vi "AlliGator Load I-m-phi Dataset.vi"(5 "Image Type":string="Image", 7 "Bkgd Image Subtraction?":bool, 8 "error in (no error)":errorcluster, 9 "Control References":T1, 10 "Folder Path":path, 11 "AlliGator IV DVR in":refnum<data-value>) -> (0 "error out":errorcluster, 2 "Folder Path (dup)":path, 3 "AlliGator IV DVR out":refnum<data-value>, 4 "Result String":string)   [LabVIEW 2021, in "AlliGator Files.lvlib"]
doc: "Loads a FLI dataset comprised of an intensity and phase image (FLIMBox)."
uses:
  AlliGator Files.lvlib
  Internal Variables/AlliGator Internal Variables v2.ctl
  <vilib>/vision/Image Controls.llb/IMAQ Image.ctl
  Internal Variables/AlliGator Gate Image Set.ctl
  AlliGator FLI Dataset Type.ctl
  AlliGator Data Series Type.ctl
  Dual-Channel Datasets/AlliGator Dataset Channel.ctl
  Settings/AlliGator Gate Arithmetic.ctl
  Source Image/AlliGator Displayed Image.ctl
  Image/Named ROI Description.ctl
  Phasor Graph/AlliGator Decay Metadata v3.ctl
  Decay Analysis/Decay Preprocessing/AlliGator Decay Background Subtraction Info.ctl
  Decay Analysis/Decay Preprocessing/AlliGator Baseline Subtraction Method.ctl
  Graphs/XY Graph/XY Graph Plot Shift Parameters.ctl
  Graphs/XY Graph/XY Graph Plot Shift Method.ctl
  Decay Analysis/Decay Preprocessing/AlliGator Decay Extrapolation Parameters.ctl
  Phasor/Calibration Phasor (m, phi).ctl
  Phasor/Phasor Reference Series.ctl
  Phasor/Phasor Calibration Map v2.ctl
  Phasor/Phasor (g, s).ctl
  Phasor Graph/AlliGator Raw Phasor Plot Data v5.ctl
  Phasor/Phasor Standard Deviation Options.ctl
  Phasor Plot/AlliGator Phasor Multi-Harmonic Data.ctl
  Phasor/Phasor Harmonic Data.ctl
  Decay Fit Parameter Map/AlliGator Decay Fit Options & Parameters v4.ctl
  Fits/IRF(X)PSED/Decay Fit Options v4.ctl
  Fits/Decay Convolution/Decay Model.ctl
  Fits/Residual Type.ctl
  Fits/IRF(X)PSED/Fit Weights Type v2.ctl
  Fits/Non-linear Fitting Method v2.ctl
  Fits/Fit Calculation Method.ctl
  Fits/Non-linear Fitting Algorithm.ctl
  Decay Analysis/Decay Fit/AlliGator Decay Fit Parameter Constraints 2.ctl
  Fits/IRF(X)PSED/Decay Fit Parameters In List.ctl
  Fits/IRF(X)PSED/MLE Baseline Offset Type.ctl
  Decay Analysis/Decay Preprocessing/AlliGator Decay Preprocessing Parameters.ctl
  Fits/IRF(X)PSED/Decay Fit Parameters & Derived Quantities List v2.ctl
  Fits/IRF(X)PSED/Decay Fit Result Constraint.ctl
  Decay Fit Parameter Map/AlliGator Parameter Maps Data.ctl
  GUI/AlliGator Dataset Ctrl Refnums.ctl
  AlliGator After Loading Dataset Information.ctl
  AlliGator ICCD-specific Information.ctl
  AlliGator I-m-phi Component List.ctl
  089290e1-c93f-4b42-a3f3-b2d44885c075.vi
  Arrays/n x n Kernel Convolution (SGL).vi
  Arrays/n x n Smoothen Array (SGL) v3.vi
  Arrays/n x n Kernel Convolution (SGL).vi/d0ebc029-cbaa-4c82-a58c-923c59c440da.vi
  Arrays/n x n Kernel Convolution (SGL).vi/b80d5e79-a0c8-46e2-aba9-3d60e0093a16.vi
  <vilib>/Analysis/2dsp.llb/Convolution.vi
  <vilib>/Analysis/2dsp.llb/2D Convolution (DBL).vi
  Arrays/Truncate Kernel.vi
  Arrays/Replace NaN by 0 (2D SGL).vi
  Arrays/n x n Smoothen Array (SGL) v3.vi/d0ebc029-cbaa-4c82-a58c-923c59c440da.vi
  Arrays/n x n Smoothen Array (SGL) v3.vi/b80d5e79-a0c8-46e2-aba9-3d60e0093a16.vi
  Arrays/Replace NaN by 0 (2D SGL).vi/df975b44-f6c5-4554-af30-980613d33749.vi
  Time/High Resolution Timing.vi
  Arrays/Compute n x n Kernel (SGL).vi
  <vilib>/Utility/error.llb/Simple Error Handler.vi
  <vilib>/Utility/error.llb/Error Cluster From Error Code.vi
  <vilib>/ErrorRing/Error Ring.xnode
  Image/Image.lvlib
  Source Image/AlliGator Source Image.lvlib
  GUI/AlliGator GUI.lvlib
  GUI/GUI.lvlib
  Boolean/Boolean.lvlib
  Error/Error.lvlib
  Arrays/Arrays.lvlib
  Strings/Strings.lvlib
  Internal Variables/AlliGator Internal Variables.lvlib
  Phasor/Phasor.lvlib
  Decay Analysis/Decay Preprocessing/AlliGator Decay Preprocessing.lvlib
  Graphs/XY Graph/XY Graph Add-Ons.lvlib
  Phasor Graph/AlliGator Phasor Graph.lvlib
  Phasor Plot/AlliGator Phasor Plot.lvlib
  Fits/Fits.lvlib
  Decay Analysis/Decay Fit/AlliGator Decay Fit.lvlib
  Settings/AlliGator Settings.lvlib
  Dual-Channel Datasets/AlliGator Dual-Channel Datasets.lvlib
  Decay Fit Parameter Map/AlliGator Decay Fit Parameter Map.lvlib
panel:
  out "# disposed images":i32
  out "# created images":i32
  # "see the AlliGator License on the block diagram (Ctrl+E or Window:Show Block Diagram)"
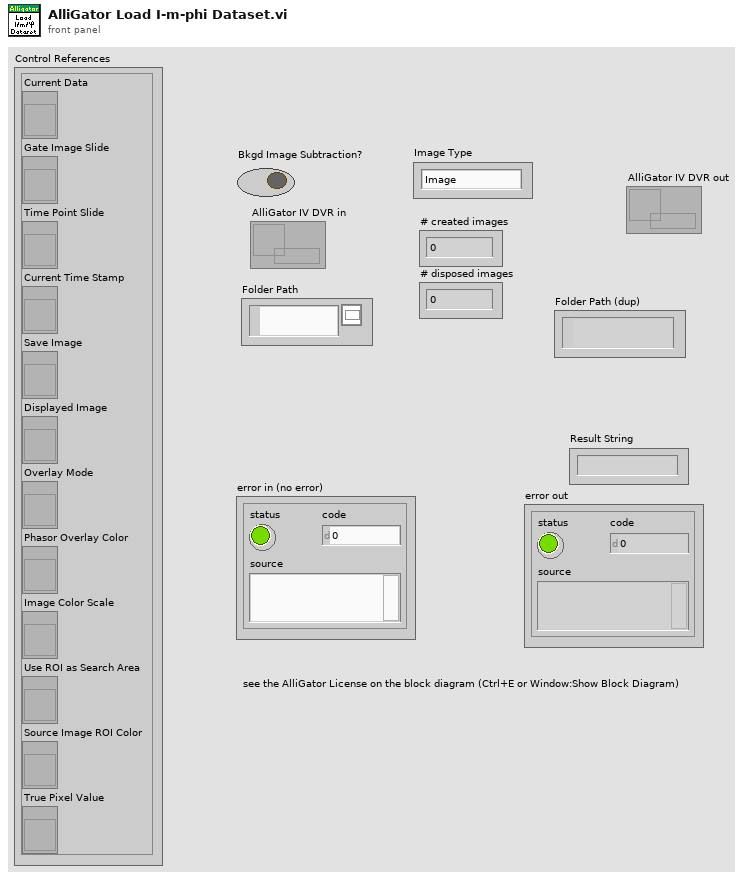
[diagram p1: front panel]
types:
  T1 = typedef "AlliGator GUI.lvlib/AlliGator Dataset Ctrl Refnums.ctl" = cluster{"Current Data":refnum<vi>, "Gate Image Slide":refnum<vi>, "Time Point Slide":refnum<vi>, "Current Time Stamp":refnum<vi>, "Save Image":refnum<vi>, "Displayed Image":refnum<vi>, "Overlay Mode":refnum<vi>, "Phasor Overlay Color":refnum<vi>, "Image Color Scale":refnum<vi>, "Use ROI as Search Area":refnum<vi>, "Source Image ROI Color":refnum<vi>, "True Pixel Value":refnum<vi>}
  T2 = typedef "AlliGator Files.lvlib/AlliGator After Loading Dataset Information.ctl" = cluster{"Nanotime Gate Separation":dbl[unit], "Gate Width":dbl[unit], "Laser Period":dbl[unit], "Data Description":string, "# Pixel X":i32, "# Pixel Y":i32, "Gates to Use":cluster{"Start":u32, "End":u32}, "Gate Step":i32, "SYNC Period":dbl[unit], "X Binning":i32, "Y Binning":i32, "Gates to":bool, "Metadata":string, "Gate Image Exposure":dbl[unit], "Gate Image Integration":dbl[unit], "Macrotime Gate Separation":dbl[unit], "ICCD-specific Information":T3}
  T3 = typedef "AlliGator Files.lvlib/AlliGator ICCD-specific Information.ctl" = cluster{"V MCP":dbl[unit], "X Hardware Binning":dbl, "Y Hardware Binning":dbl, "Gate Image Integration":dbl[unit], "Laser Power":dbl[unit]}
  T4 = typedef "AlliGator Files.lvlib/AlliGator FLI Dataset Type.ctl" = enum16{"HDF5 FLI Dataset", "Gate Image Folder", ".sdt FLI Dataset (Becker & Hickl)", ".ptu FLI Dataset (PicoQuant)", "SS1 FLI Dataset", "SS2 FLI Dataset", "I/m/phi Dataset", ".bin FLI Dataset (PicoQuant Binned)", ".bin FLI Dataset (Piccolo Binned)", ".mat FLI Dataset"}
  T5 = typedef "AlliGator Internal Variables.lvlib/AlliGator Gate Image Set.ctl" = cluster{"SGL Image Max":T6, "SGL Image Sum":T6, "SGL Gate Images":T6[], "SGL Image Min":T6}
  T6 = typedef "IMAQ Image.ctl" = refnum<image>
  T7 = typedef "AlliGator Files.lvlib/AlliGator I-m-phi Component List.ctl" = enum16{"Intensity", "g", "s"}
  T8 = typedef "FLIMBox.lvlib/FLIMbox Data.ctl" = cluster{"Software":string, "Base Frequency":dbl[unit], "X Size":i32, "Y Size":i32, "Metadata":string, "Intensity":sgl[][], "Harmonic Number":u8, "Harmonic Orders":u8[], "Harmonic Data":T9[], "File Version":string}
  T9 = typedef "FLIMBox.lvlib/FLIMbox Harmonic Data.ctl" = cluster{"Modulus":sgl[][], "Phase":sgl[][], "Harmonic Order":u8}
  T10 = typedef "AlliGator Source Image.lvlib/AlliGator Image Loading Options.ctl" = cluster{"Pixel Well Capacity":u32, "Pile-up Correction":bool, "Gate Step":i32, "Image Smoothing Options":T11, "Gates to Skip":T14, "File Background Subtraction":bool, "Background File Path":path, "Image Binning Options":T15, "# Gates":u32, "Gates to Keep":T16, "Define Gates to":bool, "Hot Pixel Removal":T17, "Dataset Scaling Factor":dbl, "Image Pre-processing Steps":T18[]}
  T11 = typedef "AlliGator Settings.lvlib/AlliGator Image Smoothing Options.ctl" = cluster{"Use Image Smoothing":bool, "Kernel Type":T12, "Bin":i32, "Algorithm":T13}
  T12 = typedef "Arrays.lvlib/Kernel Type.ctl" = enum16{"Uniform", "Bilinear", "Gaussian"}
  T13 = typedef "Arrays.lvlib/Smoothing Algorithm.ctl" = enum16{"Rapid", "Thorough"}
  T14 = typedef "AlliGator Settings.lvlib/AlliGator Background Subtraction Parameters.ctl" = cluster{"Start":u32, "End":u32}
  T15 = typedef "AlliGator Source Image.lvlib/AlliGator Image Binning Options.ctl" = cluster{"Use Image Binning":bool, "X Bin":i32, "Y Bin":i32}
  T16 = typedef "AlliGator Settings.lvlib/AlliGator Gates to Keep.ctl" = cluster{"First":u32, "Last":u32}
  T17 = typedef "SwissSPAD Live.lvlib/SwissSPAD Live_Image Display Options.ctl" = cluster{"Remove Screamers":bool, "Delta":sgl, "Equalize Histogram":bool, "Percentile":sgl, "Hot Pixel Mask Image":path, "Use Hot Pixel Mask":bool}
  T18 = typedef "AlliGator Files.lvlib/AlliGator Image Pre-processing Step.ctl" = enum16{"Remove Screamers", "Pile-up Correction", "Binning", "Smoothing", "Rescaling", "Dead Left Column Correction"}
  T19 = typedef "AlliGator Internal Variables.lvlib/AlliGator Internal Variables v2.ctl" = cluster{"----------------------------- Images -----------------------------":u8, "Displayed Image":T6, "White Light Image":T6, "Mask Image":T6, "ROI Mask Image":T6, "Current Dataset Images 1":T5, "Background Dataset Images 1":T5, "Current Dataset Images 2":T5, "Background Dataset Images 2":T5, "Current Dataset Arithmetic Images":T5, "Accumulated Dataset Images 1":T5, "Accumulated Dataset Images 2":T5, "Accumulated Dataset Arithmetic Images":T5, "----------------------------- File Paths -----------------------------":u8, "Phasor Plot Image":T6, "Decay Fit Parameter Map Image":T6, "Parameter Map Image":T6, "Single Data Point Path":path, "White Light Image Path":path, "Mask Image Path":path, "Time-Series Folder":path, "[Time-Series Paths]":path[], "----------------------------- FLI Dataset -----------------------------":u8, "Current Dataset":i32, "Single Dataset Type":T4, "Current Folder":string, "AlliGator Data Series Type":T20, "# Datasets":i32, "Dual-Channel Dataset":bool, "Selected Channel Name":string, "Dataset Channel":T21, "Channel Arithmetic":T22, "Dual-Channel Background Dataset":bool, "Background Channel":T21, "Dual-Channel Accumulated Dataset":bool, "Start Time":dbl, "[Time-Series Timestamps]":dbl[], "[Intensity Corrections]":dbl[], "Time Series Script":bool, "Type of Displayed Image":T23, "Gate Image Slide":u16, "# Gates":i32, "ROIs":T24[], "----------------------------- Decays -----------------------------":u8, "ROI Decay":cluster{"t Array":dbl[], "I Array":dbl[]}, "Valid Decay":bool, "Decay  Metadata":T26, "Reference Decay Plot Name":string, "Reference Decay":cluster{"t Array":dbl[], "I Array":dbl[]}, "Decay Shift Plot":cluster{"Time Stamps":dbl[], "Decay Shifts":dbl[]}, "[Decays Max Values]":sgl[], "[Decays Min Values]":sgl[], "----------------------------- Calibration -----------------------------":u8, "Calibration Phasor":T32, "Calibration Phasor Series":T33, "Phasor Calibration Map":T34, "Calibration Map MD5 Digest":string, "----------------------------- Phasor Graph -----------------------------":u8, "Last Raw Phasor":T35, "Last Calibrated Phasor":T35, "Last Calibrated Phasor SDV":T35, "Phasor Graph:Phasor Plot":cluster{"g Array":dbl[], "s Array":dbl[]}, "Phasor Graph:Phasor SDV Plot":cluster{"g Array":dbl[], "s Array":dbl[]}, "[Phasor Graph:Raw Phasor Plots]":T36[], "Phasor Plot locked to Ref 1":i32, "[Phasor Plot(s) locked to Ref 1]":i32[], "[Phasor Plot(s) locked to Ref 2]":i32[], "[Pixel Phasors]":T35[], "----------------------------- Phasor Plot -----------------------------":u8, "[[Sum Image]]":dbl[][], "[[CSG Phasors]]":csg[][], "[[Valid Pixel?]]":bool[][], "[[Phasor Ratios]]":dbl[][], "[[Average Lifetimes]]":dbl[][], "Amplitude Weighted Average Lifetime":bool, "I/m/phi Dataset":cluster{"I/m/phi Dataset?":bool, "Base Frequency":dbl[unit], "Harmonic Orders":u8[]}, "Multi Phasor Plot Data":T38, "----------------------------- Decay Fit Parameter Map -----------------------------":u8, "Decay Fit Options & Parameters":T40, "Fit Options: Decay Preprocessing Parameters":T51, "Fit Options: Reference Decay":cluster{"t Array":dbl[], "I Array":dbl[]}, "Is Full Image Parameters Map":bool, "Is Single-Pixels Parameters Map":bool, "NLSF Parameters Map X Resolution":i32, "NLSF Parameters Map Y Resolution":i32, "[Single Decay Fit Parameters]":dbl[], "Fit Model":T42, "[[Multiple Decays Fit Parameters]]":dbl[][], "[[Multiple Decays Fit Parameter SDVs]]":dbl[][], "[[IRFs]]":dbl[][], "[ROI Descriptors]":T25[], "IRF Array Time Axis":dbl[], "Decay Array Time Axis":dbl[], "[Decay Fit Parameter Names]":T52[], "[Decay Sum]":dbl[], "Array of Decay Fit Result Constraints":T53[], "Selected ROIs Array":bool[], "----------------------------- Parameter Maps -----------------------------":u8, "[Map Set Names]":string[], "[Parameter Maps]":T54[], "[[User-defined Quantities]]":dbl[][], "User-defined Quantity":string}
  T20 = typedef "AlliGator Files.lvlib/AlliGator Data Series Type.ctl" = enum16{"Not a Supported Series", "Gate Images Folder Series", "SwissSPAD 2 Dataset Series", "B&H FLI Dataset Series", "PicoQuant PTU FLI Dataset Series", "PicoQuant BIN FLI Dataset Series", "Piccolo hist BIN FLI Dataset Series", "HDF5 FLI Dataset Series"}
  T21 = typedef "AlliGator Dual-Channel Datasets.lvlib/AlliGator Dataset Channel.ctl" = enum16{"G2", "INT"}
  T22 = typedef "AlliGator Settings.lvlib/AlliGator Gate Arithmetic.ctl" = enum16{"None", "INT-G2", "G2/INT*<INT>", "(1 - G2/INT)*<INT>"}
  T23 = typedef "AlliGator Source Image.lvlib/AlliGator Displayed Image.ctl" = enum16{"Single Gate", "Sum of All Gates", "Max of All Gates", "Min of All Gates", "-", "White Ligth Image", "Mask Image"}
  T24 = typedef "Image.lvlib/Named ROI Description.ctl" = cluster{"ROI Descriptor":T25, "ROI Name":string, "Overlay Color":u32}
  T25 = typedef "ROI Descriptor" = cluster{"Global Rectangle":i32[], "Contours":cluster{"ID":enum32{"External", "Internal"}, "Type":u32, "Coordinates":i32[]}[]}
  T26 = typedef "AlliGator Phasor Graph.lvlib/AlliGator Decay Metadata v3.ctl" = cluster{"ROI Descriptor":T25, "ROI Center":cluster{"X":i32, "Y":i32}, "Decay Background Subtraction Info":T27, "Decay Reverted":bool, "Decay Smoothened":bool, "Decay Straightened":bool, "Fitted Tau (Decay Straightening)":dbl, "Decay Shift Parameters":T29, "Decay Shifted":bool, "Decay Extrapolated":bool, "Decay Extrapolation Parameters":T31, "Decay Normalized":bool, "Fold Decay":bool, "# Folds":u32}
  T27 = typedef "AlliGator Decay Preprocessing.lvlib/AlliGator Decay Background Subtraction Info.ctl" = cluster{"Laser Period":dbl[unit], "Gate Duration":dbl[unit], "Baseline Subtraction Method":T28, "Background Definition Range":cluster{"Min Gate":dbl[unit], "Max Gate":dbl[unit]}, "Total Intensity w/o Bkgd Subtraction":dbl, "Bkgd-subtracted Intensity (exp)":dbl, "# Data Points":i32, "Background/Gate":dbl, "Fitted Lifetime":dbl[unit], "Bkgd-subtracted Intensity (theo)":dbl}
  T28 = typedef "AlliGator Decay Preprocessing.lvlib/AlliGator Baseline Subtraction Method.ctl" = enum16{"Mean", "Min", "Square Gated Single-Exponential", "File", "Constant"}
  T29 = typedef "XY Graph Add-Ons.lvlib/XY Graph Plot Shift Parameters.ctl" = cluster{"Type":T30, "Shift":dbl[unit], "Threshold":dbl, "Rotate":bool}
  T30 = typedef "XY Graph Add-Ons.lvlib/XY Graph Plot Shift Method.ctl" = enum16{"Default", "CFD", "Threshold", "Cross-Correlation"}
  T31 = typedef "AlliGator Decay Preprocessing.lvlib/AlliGator Decay Extrapolation Parameters.ctl" = cluster{"Additional Points":u32, "Head Fraction":dbl, "Fitted Tau":dbl, "Use Periodicity":bool, "Use Cursors":bool, "Tail Fraction":dbl}
  T32 = typedef "Phasor.lvlib/Calibration Phasor (m, phi).ctl" = cluster{"m":dbl, "phi":dbl, "Phasor Frequency":dbl[unit], "Reference Lifetime":dbl[unit]}
  T33 = typedef "Phasor.lvlib/Phasor Reference Series.ctl" = cluster{"m Array":dbl[], "phi Array":dbl[], "Phasor Frequency":dbl[unit], "Calibration Lifetime":dbl[unit]}
  T34 = typedef "Phasor.lvlib/Phasor Calibration Map v2.ctl" = cluster{"Phasor Frequency":dbl[unit], "Calibration Lifetime":dbl[unit], "ROI Centers":cluster{"X":i32, "Y":i32}[], "ROI Descriptors":T25[], "Map Resolution X":i32, "Map Resolution Y":i32, "z Array":cdb[]}
  T35 = typedef "Phasor.lvlib/Phasor (g, s).ctl" = cluster{"g":dbl, "s":dbl}
  T36 = typedef "AlliGator Phasor Graph.lvlib/AlliGator Raw Phasor Plot Data v5.ctl" = cluster{"Phasor Plot Name":string, "Raw Phasor Plot":T35[], "Phasor Frequency":dbl[unit], "[Decay Metadata]":T26[], "Raw Phasor Plot SDV":T35[], "Phasor SDV Options":T37, "[Calibration Phasor]":T32[], "Intensity Array":dbl[]}
  T37 = typedef "Phasor.lvlib/Phasor Standard Deviation Options.ctl" = cluster{"Compute Estimated SDV":bool, "# Replicas":u32, "Use Estimated Average Phasor":bool}
  T38 = typedef "AlliGator Phasor Plot.lvlib/AlliGator Phasor Multi-Harmonic Data.ctl" = cluster{"Base Frequency":dbl[unit], "# Harmonics":u8, "Harmonic Orders":u8[], "Phasor Plot Settings Checksum":u64, "Phasor Harmonic Data Array":T39[]}
  T39 = typedef "Phasor.lvlib/Phasor Harmonic Data.ctl" = cluster{"Phasor Harmonic Name":string, "Phasor Plot Settings Checksum":u64, "Phasor Frequency":dbl[unit], "Base Frequency":dbl[unit], "Harmonic Order":u8, "Phasor Plot Parameters":string, "Phasor Array [[CSG]]":csg[][], "Dataset File Path":path}
  T40 = typedef "AlliGator Decay Fit Parameter Map.lvlib/AlliGator Decay Fit Options & Parameters v4.ctl" = cluster{"SYNC Period":dbl[unit], "Fit Options":T41, "Fit Parameter Constraints":T48[], "MLE Baseline Offset":dbl, "MLE Baseline Offset Type":T50}
  T41 = typedef "Fits.lvlib/Decay Fit Options v4.ctl" = cluster{"Show Fit Residuals":bool, "Fit Model":T42, "Residual Type":T43, "Max Decay Percentile":dbl, "Min Decay Percentile":dbl, "Show Full Decay":bool, "Weights":T44, "Fitting Method":T45, "Compute Parameter Uncertainties":bool, "Periodic Boundaries":bool, "Model Calculation":T46, "Period":dbl[unit], "Termination Criteria":cluster{"Max Iterations":i32, "Max Function Calls":i32, "Max Time":dbl[unit], "Function Tolerance":dbl, "Parameter Tolerance":dbl, "Gradient Tolerance":dbl, "Min Lambda":dbl, "Max Lambda":dbl, "Initial Tick Count":u32}, "Offset Resolution":dbl[unit], "Use Local IRF":bool, "Fitting Algorithm":T47, "Show Confidence Interval ":bool, "Confidence Level":dbl}
  T42 = typedef "Fits.lvlib/Decay Model.ctl" = enum16{"1-Exponential", "2-Exponentials"}
  T43 = typedef "Fits.lvlib/Residual Type.ctl" = enum16{"Standard", "Normalized", "Reduced"}
  T44 = typedef "Fits.lvlib/Fit Weights Type v2.ctl" = enum16{"Unweighted", "1/Variance (Neyman)", "1/Variance (Pearson)", "Best of All"}
  T45 = typedef "Fits.lvlib/Non-linear Fitting Method v2.ctl" = enum16{"Least Square", "Least Absolute Residual", "Bisquare", "MLE", "-", "Best of All"}
  T46 = typedef "Fits.lvlib/Fit Calculation Method.ctl" = enum16{"Simulation", "Convolution", "Integration"}
  T47 = typedef "Fits.lvlib/Non-linear Fitting Algorithm.ctl" = enum16{"Levenberg-Marquardt", "Trust-Region Dogleg"}
  T48 = typedef "AlliGator Decay Fit.lvlib/AlliGator Decay Fit Parameter Constraints 2.ctl" = cluster{"Fit Parameter":T49, "Min Value":dbl, "Max Value":dbl, "Global":bool, "Used":bool}
  T49 = typedef "Fits.lvlib/Decay Fit Parameters In List.ctl" = enum16{"Offset", "Baseline", "A_1", "tau_1", "A_2", "tau_2"}
  T50 = typedef "Fits.lvlib/MLE Baseline Offset Type.ctl" = enum32{"Absolute", "Percentage"}
  T51 = typedef "AlliGator Decay Preprocessing.lvlib/AlliGator Decay Preprocessing Parameters.ctl" = cluster{"Background Subtraction":bool, "Straighten Decay":bool, "Reverse Gates":bool, "1-Normalized Decay":bool, "Smoothen Decay":bool, "Smoothing Parameter":dbl, "Shift Decay":bool, "Decay Shift Parameters":T29, "Extrapolate Decay":bool, "Additional Points":u32, "Head Fraction":dbl, "Pixel-Normalize Decay":bool, "Use Periodicity":bool, "Use Cursors":bool, "Tail Fraction":dbl, "Use Decay Pre-Processing":bool, "Fold Decay":bool, "# Folds":u32, "[0-1]-Normalized Decay":bool}
  T52 = typedef "Fits.lvlib/Decay Fit Parameters & Derived Quantities List v2.ctl" = enum16{"Offset", "Baseline", "A_1", "tau_1", "A_2", "tau_2", "<tau>_a", "f1_a", "f2_a", "<tau>_i", "f1_i", "f2_i", "-", "R^2", "Chi^2"}
  T53 = typedef "Fits.lvlib/Decay Fit Result Constraint.ctl" = cluster{"Fit Parameter":enum16{"Offset", "Baseline", "A_1", "tau_1", "A_2", "tau_2", "<tau>_a", "f1_a", "f2_a", "<tau>_i", "f1_i", "f2_i", "-", "R^2", "Chi^2", "Max Relative Residual", "<Residual ACF>", "Residual ACF SDV", "tau_2/tau_1"}, "Min Value":dbl, "Max Value":dbl, "Use Constraint":bool}
  T54 = typedef "AlliGator Decay Fit Parameter Map.lvlib/AlliGator Parameter Maps Data.ctl" = cluster{"Map Set Name":string, "[Parameter Names]":string[], "[[Parameters]]":dbl[][], "[[Parameter SDVs]]":dbl[][], "Decay Array Time Axis":dbl[], "[[IRFs]]":dbl[][], "IRF Array Time Axis":dbl[], "X Resolution":i32, "Y Resolution":i32, "Intensity Array":dbl[]}
  T55 = typedef "Image Type" = u32
  T56 = typedef "Image.lvlib/Image Characteristics.ctl" = cluster{"Calibration":T57, "File Type":string, "X Resolution":i32, "Y Resolution":i32, "File Data Type":i32, "Image Type":T55}
  T57 = typedef "Simple Grid Descriptor" = cluster{"X Step":sgl, "Y Step":sgl, "Unit":T58}
  T58 = typedef "Image Unit" = enum32{"Undefined", "Angström", "Micrometer", "Millimeter", "Centimeter", "Meter", "Kilometer", "Microinch", "Inch", "Feet", "Nautical miles", "Standard miles", "Steps"}
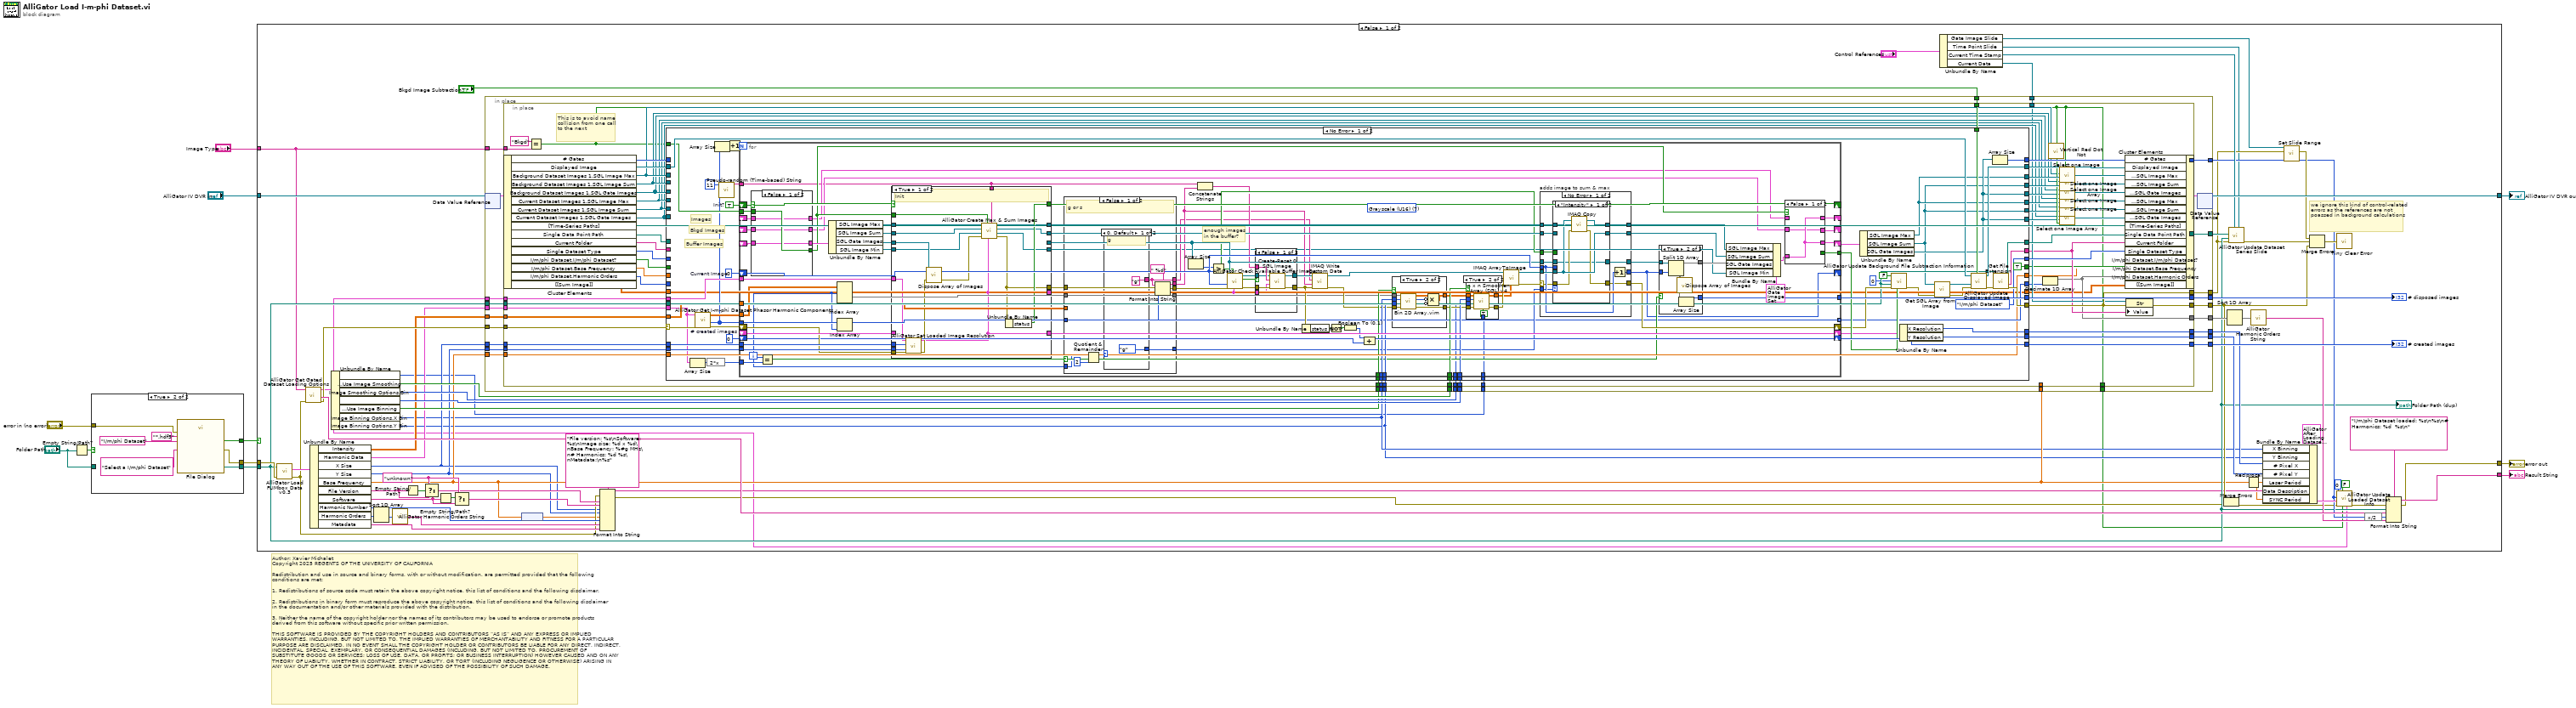
[diagram p0: block diagram]
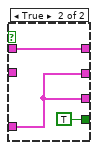
[diagram p2: hidden frame]
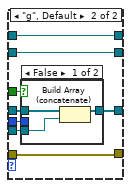
[diagram p6: hidden frame]
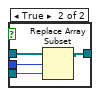
[diagram p7: hidden frame]
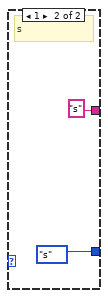
[diagram p10: hidden frame]
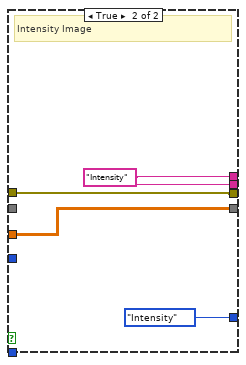
[diagram p11: hidden frame]
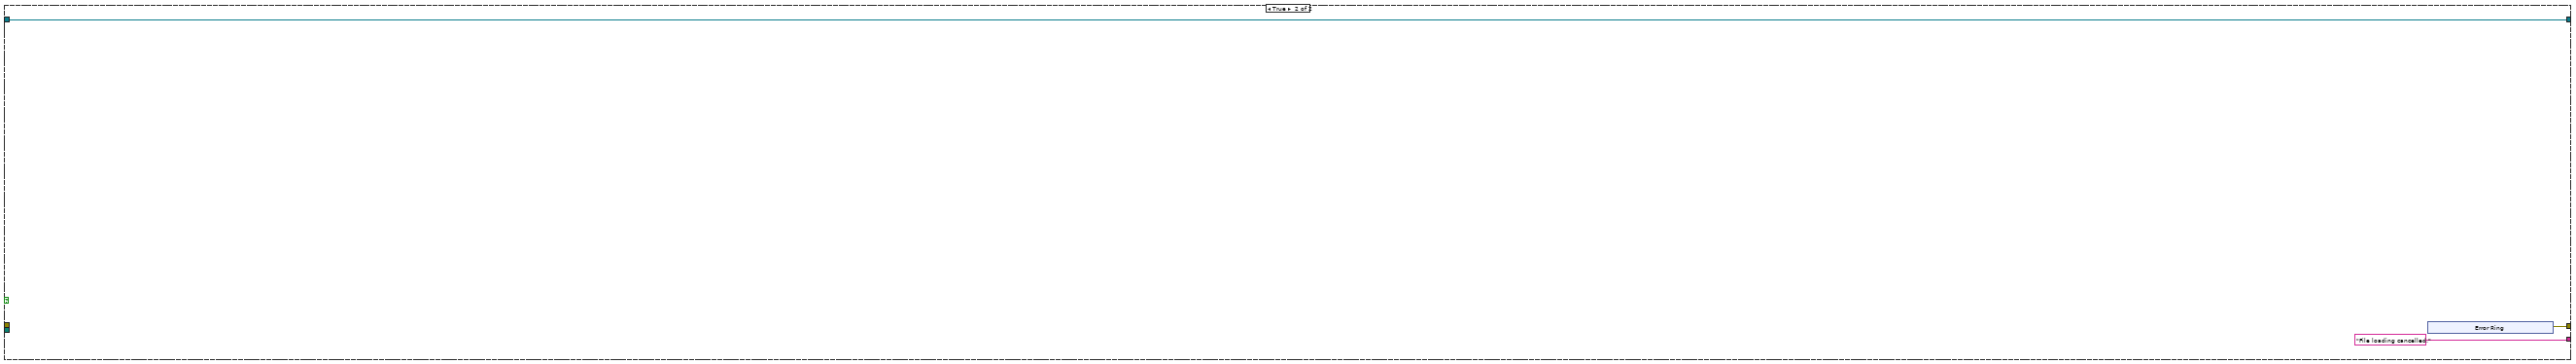
[diagram p16: hidden frame]
diagram:
  # "Author: Xavier Michalet\nCopyright 2025 REGENTS OF THE UNIVERSITY OF CALIFORNIA\n\nRedistribution and use in source and binary forms, with or without modification, are permitted provided that the following conditions are met:\n\n1. Redistributions of source code must retain the above copyright notice, this list of conditions and the following disclaimer.\n\n2. Redistributions in binary form must reproduce the above copyright notice, this list of conditions and the following disclaimer in the documentation and/or other materials provided with the distribution.\n\n3. Neither the name of the copyright holder nor the names of its contributors may be used to endorse or promote products derived from this software without specific prior written permission.\n\nTHIS SOFTWARE IS PROVIDED BY THE COPYRIGHT HOLDERS AND CONTRIBUTORS “AS IS” AND ANY EXPRESS OR IMPLIED WARRANTIES, INCLUDING, BUT NOT LIMITED TO, THE IMPLIED WARRANTIES OF MERCHANTABILITY AND FITNESS FOR A PARTICULAR PURPOSE ARE DISCLAIMED. IN NO EVENT SHALL THE COPYRIGHT HOLDER OR CONTRIBUTORS BE LIABLE FOR ANY DIRECT, INDIRECT, INCIDENTAL, SPECIAL, EXEMPLARY, OR CONSEQUENTIAL DAMAGES (INCLUDING, BUT NOT LIMITED TO, PROCUREMENT OF SUBSTITUTE GOODS OR SERVICES; LOSS OF USE, DATA, OR PROFITS; OR BUSINESS INTERRUPTION) HOWEVER CAUSED AND ON ANY THEORY OF LIABILITY, WHETHER IN CONTRACT, STRICT LIABILITY, OR TORT (INCLUDING NEGLIGENCE OR OTHERWISE) ARISING IN ANY WAY OUT OF THE USE OF THIS SOFTWARE, EVEN IF ADVISED OF THE POSSIBILITY OF SUCH DAMAGE."
  n1 = Empty String/Path?(string/path="Folder Path") -> (empty?=w7:bool)
  n2 = case shown="True" w7 {
    tunnel: "error in (no error)" -> [w12 w20]
    tunnel: [w13 w17] -> w4
    tunnel: [w12 w16] -> w3
    tunnel: "Folder Path" -> [w13 _]
    tunnel: [_ w15] -> w2
    frame False {
    }
    frame True {
      n3 = call "File Dialog"("prompt"="Select a I/m/phi Dataset", "error in"=w20, "pattern (all files)"="*.hdf5", "pattern label"="I/m/phi Dataset") -> ("selected path"=w17:path, "cancelled"=w15:bool, "error out"=w16:errorcluster)  [unwired: 8 in, 1 out]
    }
  }
  n4 = case shown="False" w2 {
    tunnel: [w88 "File loading cancelled."] -> w11
    tunnel: [w71 w478] -> w10
    tunnel: "AlliGator IV DVR in" -> [w77 w477]
    tunnel: [w76 w477] -> w8
    tunnel: w4 -> [w53 _]
    tunnel: w3 -> [w64 _]
    tunnel: "Image Type" -> [w25 _]
    frame False {
      w44 = "unknown" ("t")
      # "we ignore this kind of control-related errors as the references are not poassed in background calculations"
      n5 = call "AlliGator Load FLIMbox Data v0.3.vi"("Error In"=w64, "File Path"=w53) -> ("Error Out"=w38:errorcluster, "FLIMbox Data out"=w54:T8)  [unwired: 8 in]
      n6 = call "AlliGator Get Gated Dataset Loading Options.vi"("error in (no error)"=w38, "Image Type"=w25) -> ("error out"=w65:errorcluster, "Dataset Loading Options string"=w82:string, "Dataset Loading Options"=w22:T10)  [unwired: 6 in, 1 out]
      n7 = Unbundle By Name(w54) -> ("Intensity"=w63:sgl[][], "Harmonic Data"=w62:T9[], "X Size"=w30:i32, "Y Size"=w29:i32, "Base Frequency"=w32:dbl[unit], "File Version"=w47:string, "Software"=w45:string, "Harmonic Number"=w41:u8, "Harmonic Orders"=w50:u8[], "Metadata"=w39:string)
      n8 = Unbundle By Name(w22) -> ("Image Smoothing Options.Algorithm"=w24:T13, "Image Smoothing Options.Use Image Smoothing"=w79:bool, "Image Smoothing Options.Bin"=w81:i32, "Image Smoothing Options.Kernel Type"=w80:T12, "Image Binning Options.Use Image Binning"=w78:bool, "Image Binning Options.X Bin"=w27:i32, "Image Binning Options.Y Bin"=w26:i32)
      n9 = Sort 1D Array(array=w50) -> (sorted array=w51:u8[])
      n10 = call "AlliGator Harmonic Orders String.vi"("Harmonic Order Array"=w51) -> ("String"=w40:string)  [unwired: 8 in]
      n11 = Empty String/Path?(string/path=w47) -> (empty?=w48:bool)
      n12 = Select(t=w44, s=w48, f=w47) -> (s? t:f=w43:string)
      n13 = Empty String/Path?(string/path=w45) -> (empty?=w46:bool)
      n14 = Select(t=w44, s=w46, f=w45) -> (s? t:f=w42:string)
      n15 = node(w32) -> (w31:dbl)
      n16 = Format Into String(format string="File version: %s\nSoftware: %s\nImage size: %d x %d\nBase Frequency: %#g MHz\n# Harmonics: %d %s\nMetadata:\n%s", error in=w38, w43, w42, w30, w29, w31, w41, w40, w39) -> (resulting string=w33:string, error out=w37:errorcluster)  [unwired: 1 in]
      n17 = Unbundle By Name("Control References") -> ("Gate Image Slide"=w73:refnum<vi>, "Time Point Slide"=w21:refnum<vi>, "Current Time Stamp"=w74:refnum<vi>, "Current Data"=w68:refnum<vi>)
      n18 = in-place {
        in-place-border: [w121] -> w90
        in-place-border: w25 -> [w120]
        in-place-border: [w119] -> w87
        in-place-border: [w118] -> w61
        in-place-border: [w117] -> w60
        in-place-border: w65 -> [w116]
        in-place-border: "Bkgd Image Subtraction?" -> [w115]
        in-place-border: [w114] -> w66
        in-place-border: w81 -> [w113]
        in-place-border: w80 -> [w112]
        in-place-border: w79 -> [w111]
        in-place-border: [w110] -> w36
        in-place-border: w78 -> [w109]
        in-place-border: w27 -> [w108]
        in-place-border: w26 -> [w107]
        in-place-border: w22 -> [w106]
        in-place-border: [w96] -> w72
        in-place-border: w68 -> [w103]
        in-place-border: [w102] -> w35
        in-place-border: w63 -> [w101]
        in-place-border: w62 -> [w100]
        in-place-border: w30 -> [w99]
        in-place-border: w29 -> [w98]
        in-place-border: w53 -> [w97]
        in-place-border: w32 -> [w95]
        in-place-border: w32 -> [w94]
        in-place-border: [w93] -> w55
        in-place-border: w24 -> [w92]
        in-place-border: [w91] -> w23
        n19 = in-place-dvr #1(w77) -> (w105:T19)  [unwired: 1 out]
        n20 = in-place {
          in-place-border: [w186] -> w121
          in-place-border: w120 -> [w163]
          in-place-border: [w185] -> w119
          in-place-border: [w184] -> w118
          in-place-border: [w183] -> w117
          in-place-border: w116 -> [w182]
          in-place-border: w115 -> [w181]
          in-place-border: [w173] -> w114
          in-place-border: w113 -> [w180]
          in-place-border: w112 -> [w179]
          in-place-border: w111 -> [w178]
          in-place-border: [w143] -> w110
          in-place-border: w109 -> [w177]
          in-place-border: w108 -> [w176]
          in-place-border: w107 -> [w175]
          in-place-border: w106 -> [w174]
          in-place-border: w103 -> [w142]
          in-place-border: [w140] -> w102
          in-place-border: w101 -> [w139]
          in-place-border: w100 -> [w138]
          in-place-border: w99 -> [w137]
          in-place-border: w98 -> [w136]
          in-place-border: w97 -> [w135]
          in-place-border: [w134] -> w96
          in-place-border: w95 -> [_]
          in-place-border: w94 -> [w128]
          in-place-border: [w126] -> w93
          in-place-border: w92 -> [w125]
          in-place-border: [w122] -> w91
          # "This is to avoid name collision from one call to the next"
          n21 = in-place-cluster #2(w105) -> ("# Gates"=w171:i32, "Displayed Image"=w170:T6, "Background Dataset Images 1.SGL Image Max"=w149:T6, "Background Dataset Images 1.SGL Image Sum"=w148:T6, "Background Dataset Images 1.SGL Gate Images"=w147:T6[], "Current Dataset Images 1.SGL Image Max"=w146:T6, "Current Dataset Images 1.SGL Image Sum"=w145:T6, "Current Dataset Images 1.SGL Gate Images"=w144:T6[], "[Time-Series Paths]"=w134:path[], "Single Data Point Path"=w168:path, "Current Folder"=w167:string, "Single Dataset Type"=w166:T4, "I/m/phi Dataset.I/m/phi Dataset?"=w132:bool, "I/m/phi Dataset.Base Frequency"=w131:dbl[unit], "I/m/phi Dataset.Harmonic Orders"=w130:u8[], "[[Sum Image]]"=w124:dbl[][])
          n22 = Equal?(x="Bkgd", y=w163) -> (x = y?=w122:bool)
          n23 = case shown="No Error" w182 {
            selector: w182 -> [w203 w474]
            tunnel: [w240 _] -> w186
            tunnel: w122 -> [w217 _]
            tunnel: [w239 _] -> w185
            tunnel: [w238 _] -> w184
            tunnel: [w237 _] -> w183
            tunnel: w181 -> [w235 _]
            tunnel: [w231 w476] -> w173
            tunnel: w180 -> [w230 _]
            tunnel: w179 -> [w229 _]
            tunnel: w178 -> [w228 _]
            tunnel: [w220 w474] -> w143
            tunnel: w177 -> [w227 _]
            tunnel: w176 -> [w226 _]
            tunnel: w175 -> [w225 _]
            tunnel: w174 -> [w224 _]
            tunnel: [w223 w475] -> w172
            tunnel: w171 -> [_ w476]
            tunnel: w170 -> [w222 w475]
            tunnel: [w219 w472] -> w169
            tunnel: [w214 w473] -> w141
            tunnel: w168 -> [_ w472]
            tunnel: w167 -> [_ w473]
            tunnel: w166 -> [_ w471]
            tunnel: [AlliGator_FLI_Dataset_Type."I/m/phi Dataset" ("Single Dataset Type") w471] -> w165
            tunnel: [w215 w470] -> w159
            tunnel: [w191 w469] -> w156
            tunnel: [w216 w468] -> w153
            tunnel: [w216 w465] -> w152
            tunnel: [w191 w466] -> w151
            tunnel: [w215 w467] -> w150
            tunnel: w149 -> [_ w470]
            tunnel: w148 -> [_ w469]
            tunnel: w147 -> [_ w468]
            tunnel: w146 -> [_ w467]
            tunnel: w145 -> [_ w466]
            tunnel: w144 -> [_ w465]
            tunnel: w139 -> [w205 _]
            tunnel: w138 -> [w198 _]
            tunnel: w137 -> [w211 _]
            tunnel: w136 -> [w210 _]
            tunnel: w135 -> [w209 _]
            tunnel: [w208 w462] -> w127
            tunnel: [TRUE ("I/m/phi Dataset.I/m/phi Dataset?") w464] -> w133
            tunnel: w132 -> [_ w464]
            tunnel: w131 -> [_ w463]
            tunnel: w130 -> [_ w462]
            tunnel: [w206 w463] -> w129
            tunnel: w128 -> [w206 _]
            tunnel: w125 -> [w197 _]
            tunnel: w124 -> [w195 w461]
            tunnel: [w194 w461] -> w123
            frame No Error {
              w241 = 0  # # created images
              w242 = 0  # Current Image
              w243 = TRUE  # Init?
              # "Images"
              # "Bkgd Images"
              # "Buffer Images"
              n24 = Array Size(array=w198) -> (size(s)=w213:i32)
              n25 = call "AlliGator Get I-m-phi Dataset Phasor Harmonic Components.vi"("Error In"=w203, "Harmonic Data"=w198) -> ("Error Out"=w202:errorcluster, "Harmonic Order"=w201:u8[], "Phasor Components"=w204:sgl[][][])  [unwired: 7 in]
              n26 = expression code="2*x"(w213) -> (w212:i32)
              n27 = Array Size(array=w201) -> (size(s)=w200:i32)
              n28 = call "Pseudo-random (Time-based) String.vi"("Length (10)"=u32 11) -> ("result string"=w196:string)  [unwired: 9 in, 1 out]
              n29 = Increment(x=w200) -> (x+1=w199:i32)
              n30 = for {
                N: w199 -> [_]
                shift-right: [w258] -> w232
                shift-left: w202 -> [w287]
                shift-right: [w311] -> _
                shift-left: _ -> [w321]
                shift-right: [w310] -> _
                shift-left: w243 -> [w322]
                shift-right: [w246] -> _
                shift-left: w242 -> [w325]
                shift-right: [w324] -> w240
                shift-left: w241 -> [w264]
                tunnel: w217 -> [w317]
                shift-right: [w313] -> w236
                shift-left: _ -> [w319]
                shift-right: [w312] -> _
                shift-left: _ -> [w320]
                tunnel: w196 -> [w248]
                tunnel: w212 -> [w323]
                tunnel: [w314] -> w239
                tunnel: [w307] -> w234
                shift-right: [w306] -> w233
                shift-left: _ -> [w305]
                tunnel: w230 -> [w250]
                tunnel: w229 -> [w302]
                tunnel: w228 -> [w301]
                tunnel: w227 -> [w300]
                tunnel: w226 -> [w299]
                tunnel: w225 -> [w298]
                tunnel: w224 -> [w297]
                tunnel: w205 -> [w269]
                tunnel: w211 -> [w289]
                tunnel: w210 -> [w288]
                tunnel: [w252] -> w208 mode=indexing
                tunnel: w204 -> [w255]
                tunnel: w201 -> [w257]
                tunnel: w197 -> [w249]
                i -> [w251]
                (unwired) T55 7 items=["Grayscale (U8)", "Grayscale (I16)", "Grayscale (SGL)", "Complex (CSG)", "RGB (U32)", "HSL (U32)", "RGB (U64)", "Grayscale (U16)"] ("Image Type")
                # "enough images in the buffer?"
                n31 = case shown="False" w322 {
                  tunnel: w317 -> [w450 w456]
                  tunnel: [w450 w456] -> w304
                  tunnel: w321 -> [w449 w453]
                  tunnel: w320 -> [w448 w454]
                  tunnel: w319 -> [w447 _]
                  tunnel: [w449 w452] -> w271
                  tunnel: [w448 w451] -> w272
                  tunnel: [w447 w455] -> w318
                  frame False {
                  }
                  frame True {
                    n32 = case shown="False" w456 {
                      tunnel: [w458 w459] -> w455
                      tunnel: w454 -> [w457 w459]
                      tunnel: w453 -> [w458 w460]
                      tunnel: [w458 w460] -> w452
                      tunnel: [w457 w459] -> w451
                      frame False {
                      }
                      frame True {
                      }
                    }
                  }
                }
                n33 = Equal?(x=w251, y=w323) -> (x = y?=w256:bool)
                n34 = Unbundle By Name(w318) -> ("SGL Image Max"=w296:T6, "SGL Image Sum"=w295:T6, "SGL Gate Images"=w292:T6[], "SGL Image Min"=w247:T6)
                n35 = Index Array(array=w255, index (dim 0)=w251) -> (element=w253:sgl[][])  [unwired: 2 in]
                n36 = Index Array(array=w257, index=w251) -> (element=w252:u8)
                n37 = case shown="True" w322 {
                  selector: w322 -> [_ w446]
                  tunnel: [w426 w444] -> w294
                  tunnel: w287 -> [w437 w442]
                  tunnel: [w439 w446] -> w310
                  tunnel: [w427 w445] -> w293
                  tunnel: w304 -> [w429 _]
                  tunnel: w296 -> [w432 w445]
                  tunnel: w295 -> [w431 w444]
                  tunnel: [w428 w441] -> w290
                  tunnel: w305 -> [_ w441]
                  tunnel: [w424 w442] -> w268
                  tunnel: w292 -> [w438 w443]
                  tunnel: [_ w443] -> w291
                  tunnel: w297 -> [w436 _]
                  tunnel: [w428 w441] -> w306
                  tunnel: w289 -> [w435 _]
                  tunnel: w288 -> [w434 _]
                  tunnel: w248 -> [w430 _]
                  tunnel: w247 -> [w423 w440]
                  tunnel: [w422 w440] -> w245
                  frame True {
                    # "Init"
                    n38 = call "AlliGator Set Loaded Image Resolution.vi"("Error In"=w437, "Image Y"=w434, "Image X"=w435, "Image Loading Options"=w436) -> ("Error Out"=w433:errorcluster, "Image Characteristics"=w428:T56)  [unwired: 6 in]
                    n39 = call "Dispose Array of Images.vi"("Array of Images"=w438, "error in (no error)"=w433) -> ("error out"=w425:errorcluster)  [unwired: 7 in]
                    n40 = call "AlliGator Create Max & Sum Images.vi"("Prefix"=w430, "Image Characteristics"=w428, "Image Type"=w429, "Error In"=w425, "Image Min"=w423, "Image Max"=w431, "Image Sum"=w432) -> ("Error Out"=w424:errorcluster, "Image Min"=w422:T6, "Image Max"=w426:T6, "Image Sum"=w427:T6)  [unwired: 1 in]
                    n41 = Unbundle By Name(w424) -> ("status"=w439:bool)
                  }
                  frame False {
                  }
                }
                n42 = case shown="False" w256 {
                  tunnel: [w411 w421] -> w261
                  tunnel: w252 -> [w409 _]
                  tunnel: [w408 w421] -> w262
                  tunnel: w268 -> [w407 w420]
                  tunnel: [w406 w420] -> w267
                  tunnel: w269 -> [_ w419]
                  tunnel: [w405 AlliGator_I-m-phi_Component_List."Intensity"] -> w260
                  tunnel: w251 -> [w404 _]
                  tunnel: w253 -> [w403 _]
                  tunnel: [w403 w419] -> w254
                  frame False {
                    # "g or s"
                    n43 = Quotient & Remainder(x=w404, y=2) -> (x-y*floor(x/y)=w412:i32)  [unwired: 1 out]
                    n44 = case shown="0, Default" w412 {
                      tunnel: ["g" ("Key") "s" ("Key")] -> w411
                      tunnel: [AlliGator_I-m-phi_Component_List."g" AlliGator_I-m-phi_Component_List."s"] -> w405
                      frame 0, Default {
                        # "g"
                      }
                      frame 1 {
                        # "s"
                      }
                    }
                    n45 = Format Into String(format string=" %d", initial string=w411, error in=w407, w409) -> (resulting string=w408:string, error out=w406:errorcluster)
                  }
                  frame True {
                    w421 = "Intensity" ("Key")
                    # "Intensity Image"
                  }
                }
                n46 = Array Size(array=w291) -> (size(s)=w286:i32)
                n47 = Concatenate Strings(w248, w262) -> (w279:string)
                n48 = Greater?(x=w286, y=w325) -> (0:w285:bool)
                n49 = call "AlliGator Check Available Buffer Image.vi"("Image Characteristics"=w290, "Buffer Image available?"=w285, "error in (no error)"=w267, "Current Gate"=w325, "Image Buffer"=w291) -> ("error out"=w275:errorcluster, "Image Reused?"=w277:bool, "Gate Image"=w278:T6)  [unwired: 3 in, 1 out]
                n50 = case shown="False" w277 {
                  tunnel: w279 -> [w400 _]
                  tunnel: w278 -> [w399 w402]
                  tunnel: [w398 w402] -> w276
                  tunnel: w275 -> [w397 w401]
                  tunnel: [w396 w401] -> w266
                  tunnel: w290 -> [w395 _]
                  frame False {
                    n51 = call "Create-Reset 0 SGL Image.vi"("Error In"=w397, "Image Characteristics"=w395, "Image Name"=w400, "Image"=w399) -> ("Error Out"=w396:errorcluster, "New Image"=w398:T6)  [unwired: 6 in]
                  }
                  frame True {
                  }
                }
                n52 = Unbundle By Name(w266) -> ("status"=w274:bool)
                n53 = call "IMAQ Write Custom Data"("error in (no error)"=w266, "Custom Data In"=w262, "Key"=w261, "Image"=w276) -> ("error out"=w265:errorcluster, "Image Out"=w270:T6)  [unwired: 6 in]
                n54 = Not(x=w274) -> (.not. x?=w273:bool)
                n55 = Boolean To (0,1)(Boolean=w273) -> (0, 1=w263:i16)
                n56 = Compound Arithmetic op=ADD(w263, w264) -> (w324:i32)
                n57 = case shown="True" w300 {
                  tunnel: w265 -> [w347 w355]
                  tunnel: [w347 w354] -> w284
                  tunnel: w299 -> [_ w350]
                  tunnel: w298 -> [_ w349]
                  tunnel: w254 -> [w348 w353]
                  tunnel: [w348 w351] -> w283
                  frame False {
                  }
                  frame True {
                    n58 = call "Bin 2D Array.vim"("Error In"=w355, "Y Bin (1)"=w349, "X Bin (1)"=w350, "Array"=w353) -> ("Error Out"=w354:errorcluster, "Binned Array"=w352:sgl[][])  [unwired: 2 in, 4 out]
                    n59 = Compound Arithmetic op=MULTIPLY(w352, invert w350, invert w349) -> (w351:dbl[][])
                  }
                }
                n60 = case shown="True" w301 {
                  tunnel: w284 -> [w337 w346]
                  tunnel: [w337 w345] -> w282
                  tunnel: [w338 w344] -> w281
                  tunnel: w283 -> [w338 w343]
                  tunnel: w302 -> [_ w341]
                  tunnel: w250 -> [_ w340]
                  tunnel: w249 -> [_ w339]
                  frame False {
                  }
                  frame True {
                    n61 = call "n x n Smoothen Array (SGL) v4.vi"("Average"=TRUE, "Algorithm"=w339, "Error In"=w346, "Kernel Size"=w340, "Kernel Type"=w341, "Array in"=w343) -> ("Error Out"=w345:errorcluster, "Array out"=w344:sgl[][])  [unwired: 3 in, 1 out]
                  }
                }
                n62 = call "IMAQ ArrayToImage"("Image Pixels (Float)"=w281, "error in (no error)"=w282, "Image"=w270) -> ("error out"=w259:errorcluster, "Image Out"=w280:T6)  [unwired: 7 in]
                n63 = case "adds image to sum & max" shown="No Error" w259 {
                  selector: w259 -> [w357 w390]
                  tunnel: w294 -> [w361 w394]
                  tunnel: [w360 w394] -> w308
                  tunnel: w280 -> [w366 _]
                  tunnel: w285 -> [w368 _]
                  tunnel: w291 -> [w367 w393]
                  tunnel: w325 -> [w364 w392]
                  tunnel: [w365 w393] -> w316
                  tunnel: [w363 w392] -> w246
                  tunnel: w293 -> [w358 w391]
                  tunnel: [w359 w391] -> w309
                  tunnel: w260 -> [w362 _]
                  tunnel: [w356 w390] -> w258
                  frame No Error {
                    n64 = case shown="\"Intensity\"" w362 {
                      tunnel: w368 -> [_ w382]
                      tunnel: w367 -> [w369 w381]
                      tunnel: w366 -> [w374 w380]
                      tunnel: [w369 w379] -> w365
                      tunnel: w364 -> [_ w378]
                      tunnel: w361 -> [_ w376]
                      tunnel: [w374 w376] -> w360
                      tunnel: [w370 w377] -> w359
                      tunnel: w358 -> [w373 w377]
                      tunnel: w357 -> [w372 w375]
                      tunnel: [w371 w375] -> w356
                      frame "Intensity" {
                        n65 = call "IMAQ Copy"("error in (no error)"=w372, "Image Dst"=w373, "Image Src"=w374) -> ("error out"=w371:errorcluster, "Image Dst Out"=w370:T6)  [unwired: 3 in]
                      }
                      frame "g", Default {
                        n66 = case shown="False" w382 {
                          tunnel: w381 -> [w385 w389]
                          tunnel: w380 -> [w384 w388]
                          tunnel: w378 -> [_ w386]
                          tunnel: [w383 w387] -> w379
                          frame False {
                            n67 = Build Array (concatenate)(w385, w384) -> (w383:T6[])
                          }
                          frame True {
                            n68 = Replace Array Subset(array=w389, new element=w388, index=w386) -> (w387:T6[])
                          }
                        }
                      }
                    }
                    n69 = Increment(x=w364) -> (x+1=w363:i32)
                  }
                  frame Error {
                  }
                }
                n70 = case shown="True" w256 {
                  tunnel: w316 -> [w331 w336]
                  tunnel: [w331 w334] -> w315
                  tunnel: w246 -> [_ w335]
                  tunnel: [_ w332] -> w314
                  frame False {
                  }
                  frame True {
                    n71 = Split 1D Array(array=w336, index=w335) -> (first subarray=w334:T6[], second subarray=w333:T6[])
                    n72 = call "Dispose Array of Images.vi"("Array of Images"=w333) -> ()  [unwired: 8 in, 1 out]
                    n73 = Array Size(array=w333) -> (size(s)=w332:i32)
                  }
                }
                n74 = Bundle By Name(cluster=T5 {"SGL Image Max"=refnum, "SGL Image Sum"=refnum, "SGL Gate Images"=[], "SGL Image Min"=refnum} ("Gate Image Set"), "SGL Image Max"=w309, "SGL Image Sum"=w308, "SGL Gate Images"=w315, "SGL Image Min"=w245) -> (w303:T5)
                n75 = case shown="False" w304 {
                  tunnel: [_ TRUE ("Init?")] -> w307
                  tunnel: [w326 w328] -> w312
                  tunnel: w303 -> [w327 w328]
                  tunnel: [w327 w329] -> w311
                  tunnel: w271 -> [_ w329]
                  tunnel: [w327 w328] -> w313
                  tunnel: w272 -> [w326 _]
                  frame False {
                  }
                  frame True {
                  }
                }
              }
              n76 = Unbundle By Name(w236) -> ("SGL Image Max"=w215:T6, "SGL Image Sum"=w191:T6, "SGL Gate Images"=w216:T6[])
              n77 = call "AlliGator Update Background File Subtraction Information.vi"("Background subtracted"=w234, "Error In"=w232, "Background Dataset Path"=w209, "Background Pixel Well Capacity"=u32 0, "Background Pile-up Correction"=FALSE) -> ("Error Out"=w193:errorcluster)  [unwired: 6 in]
              n78 = Unbundle By Name(w233) -> ("X Resolution"=w238:i32, "Y Resolution"=w237:i32)
              n79 = call "Get SGL Array from Image.vi"("error in (no error)"=w193, "Image Array in (Empty)"=w195, "Image Refnum in"=w191) -> ("error out"=w192:errorcluster, "Image Array out"=w194:dbl[][], "Image Refnum dup"=w190:T6)  [unwired: 6 in]
              n80 = call "AlliGator Update Displayed Image.vi"("Bkgd Image Subtraction?"=w235, "Error In"=w192, "Sum Image Ref"=w190, "Displayed Image Ref"=w222) -> ("Error Out"=w221:errorcluster, "Displayed Image Ref"=w223:T6)  [unwired: 6 in]
              n81 = Array Size(array=w216) -> (size(s)=w231:i32)
              n82 = call <vilib>:"Get File Extension.vi"("error in (no error)"=w221, "file"=w209) -> ("error out"=w220:errorcluster, "filename without extension"=w214:string, "dup file"=w219:path)  [unwired: 5 in, 2 out]
            }
            frame Error {
            }
          }
          n83 = Decimate 1D Array(w127) -> (w126:u8[])  [unwired: 1 out]
          n84 = call "Vertical Red Dot Not.vi"("B"=w122) -> ("Not(B)"=w154:bool)  [unwired: 8 in]
          n85 = call "Select one Image.vi"("Previous Image (F)"=w149, "New Image (T)"=w159, "Image to use"=w122) -> ("Selected Image"=w162:T6)  [unwired: 4 in]
          n86 = call "Select one Image.vi"("Previous Image (F)"=w148, "New Image (T)"=w156, "Image to use"=w122) -> ("Selected Image"=w161:T6)  [unwired: 4 in]
          n87 = call "Select one Image Array.vi"("Previous Images (F)"=w147, "New Images (T)"=w153, "Image to use"=w122) -> ("Selected Images"=w160:T6[])  [unwired: 4 in]
          n88 = call "Select one Image.vi"("Previous Image (F)"=w146, "New Image (T)"=w150, "Image to use"=w154) -> ("Selected Image"=w158:T6)  [unwired: 4 in]
          n89 = call "Select one Image.vi"("Previous Image (F)"=w145, "New Image (T)"=w151, "Image to use"=w154) -> ("Selected Image"=w157:T6)  [unwired: 4 in]
          n90 = call "Select one Image Array.vi"("Previous Images (F)"=w144, "New Images (T)"=w152, "Image to use"=w154) -> ("Selected Images"=w155:T6[])  [unwired: 4 in]
          n91 = in-place-cluster #2("# Gates"=w173, "Displayed Image"=w172, "Background Dataset Images 1.SGL Image Max"=w162, "Background Dataset Images 1.SGL Image Sum"=w161, "Background Dataset Images 1.SGL Gate Images"=w160, "Current Dataset Images 1.SGL Image Max"=w158, "Current Dataset Images 1.SGL Image Sum"=w157, "Current Dataset Images 1.SGL Gate Images"=w155, "[Time-Series Paths]"=w134, "Single Data Point Path"=w169, "Current Folder"=w141, "Single Dataset Type"=w165, "I/m/phi Dataset.I/m/phi Dataset?"=w133, "I/m/phi Dataset.Base Frequency"=w129, "I/m/phi Dataset.Harmonic Orders"=w126, "[[Sum Image]]"=w123) -> (w104:T19)
          n92 = property class="Str"(reference=w142, error in=w143, "Value"=w141) -> (error out=w140:errorcluster)  [unwired: 1 out]
        }
        n93 = in-place-dvr #1(w104) -> (w76:refnum<data-value>)  [unwired: 1 out]
      }
      "# created images" <- w90
      "# disposed images" <- w87
      n94 = Merge Errors(w35, w37) -> (w34:errorcluster)
      n95 = Sort 1D Array(array=w55) -> (sorted array=w52:u8[])
      n96 = call "AlliGator Update Dataset Series Slide.vi"("Dataset Series Slide Ref"=w21, "Current Time Stamp Ref"=w74, "Error In"=w36, "Path"=w53, "Dataset Series Paths"=w72) -> ("Error Out"=w70:errorcluster)  [unwired: 5 in, 1 out]
      n97 = Reciprocal(x=w32) -> (1/x=w28:dbl[unit])
      n98 = call "AlliGator Harmonic Orders String.vi"("Harmonic Order Array"=w52) -> ("String"=w59:string)  [unwired: 8 in]
      n99 = Bundle By Name(cluster=T2 {"Nanotime Gate Separation"=nan, "Gate Width"=nan, "Laser Period"=nan, "Data Description"="", "# Pixel X"=-1, "# Pixel Y"=-1, "Gates to Use"={"Start"=0, "End"=0}, "Gate Step"=-1, "SYNC Period"=0.0, "X Binning"=0, "Y Binning"=0, "Gates to"=FALSE, "Metadata"="", "Gate Image Exposure"=0.0, "Gate Image Integration"=0.0, "Macrotime Gate Separation"=0.0, "ICCD-specific Information"={"V MCP"=0.0, "X Hardware Binning"=0.0, "Y Hardware Binning"=0.0, "Gate Image Integration"=0.0, "Laser Power"=0.0}}, "X Binning"=w27, "Y Binning"=w26, "# Pixel X"=w61, "# Pixel Y"=w60, "Laser Period"=w28, "Data Description"=w33, "SYNC Period"=w28) -> (w85:T2)
      n100 = call "Set Slide Range.vi"("Max"=w66, "error in (no error)"=w36, "Slide in"=w73) -> ("error out"=w69:errorcluster)  [unwired: 8 in]
      n101 = Merge Errors(w69, w70, w35) -> (w67:errorcluster)
      n102 = call "Tiny Clear Error.vi"("Error In"=w67) -> ()  [unwired: 8 in, 1 out]
      n103 = call "AlliGator Update Loaded Dataset Info.vi"("Image Loading Options"=w22, "Background File?"=w23, "Pile-up Correction"=FALSE, "error in (no error)"=w34, "After Loading Dataset Information"=w85, "# Gates"=w66, "Pixel Well Capacity"=u32 0) -> ("Error Out"=w84:errorcluster)  [unwired: 4 in]
      n104 = expression code="x/2"(w66) -> (w56:i32)
      n105 = Format Into String(format string="I/m/phi Dataset loaded: %s\n%s\n# Harmonics: %d  %s\n", error in=w84, w53, w82, w56, w59) -> (resulting string=w88:string, error out=w71:errorcluster)  [unwired: 1 in]
      "Folder Path (dup)" <- w53
    }
    frame True {
      n106 = xnode "Error Ring"() -> ("error out"=w478:errorcluster)
    }
  }
  "error out" <- w10
  "Result String" <- w11
  "AlliGator IV DVR out" <- w8
